vi "Warning.vi"(4 "Message":string, 6 "Source":string, 7 "Logger Name (Logger)":string="Logger", 8 "error in (no error)":errorcluster) -> (0 "error out":errorcluster)   [LabVIEW 2024, in "RQMHLogSingleton.lvlib"]
uses:
  RQMHLogSingleton.lvlib
  RQMHLogger/RQMHLogger.lvclass
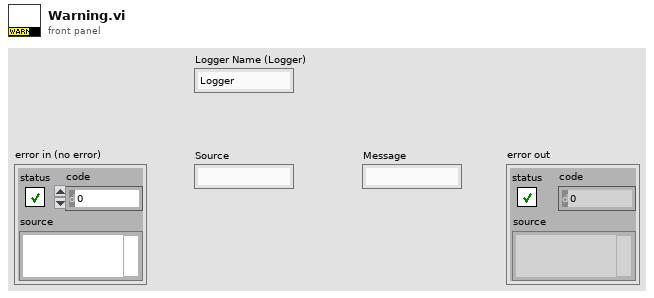
[diagram p1: front panel]
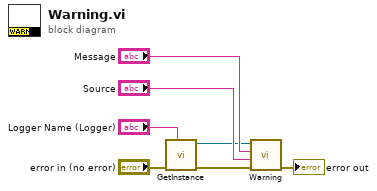
[diagram p0: block diagram]
diagram:
  n1 = call "GetInstance.vi"("Logger Name (Logger)"="Logger Name (Logger)", "error in (no error)"="error in (no error)") -> ("error out"=w2:errorcluster, "RQMHLogger Get"=w1:refnum<class "RQMHLogger.lvclass">)  [unwired: 8 in]
  n2 = call "Warning.vi"("error in (no error)"=w2, "Source"="Source", "Message"="Message", "RQMHLogger in"=w1) -> ("error out"=→"error out":errorcluster)  [unwired: 6 in, 1 out]
